vi "Filter OPC-UA-Items.vi"() -> ()   [LabVIEW 2016]
panel:
  out "Founf OPC Items":string[](array[string])
  out "found":i32
  in  "regular expression":string
  in  "sorted array":T1(array[cluster])
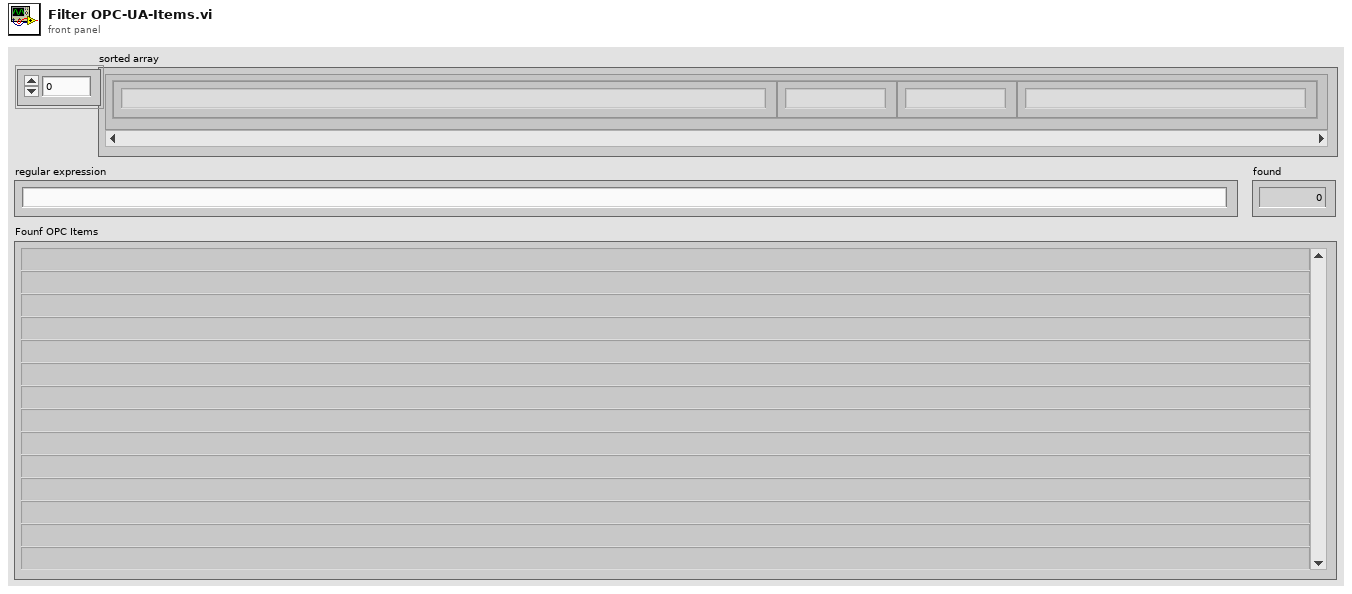
[diagram p1: front panel]
types:
  T1 = cluster{"node name":string, "String":string, "String":string, "node path":string}[]
  T2 = enum16{"open", "replace", "create", "open or create", "replace or create", "replace or create with confirmation"}
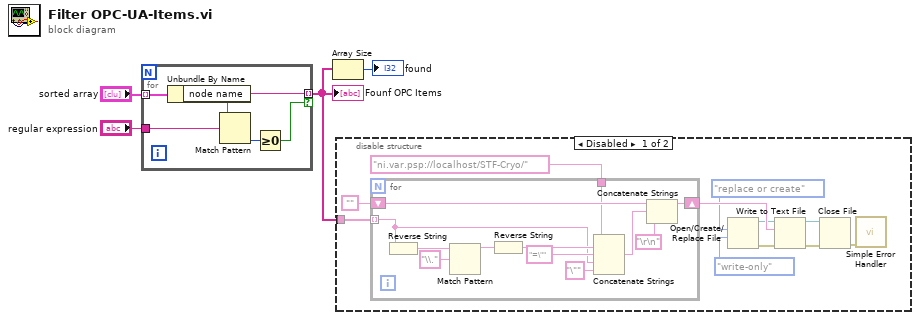
[diagram p0: block diagram]
diagram:
  n1 = for {
    tunnel: "sorted array" -> [w9] mode=indexing
    tunnel: "regular expression" -> [w8]
    tunnel: [w7] -> w1 mode=indexing if=w5
    n2 = Unbundle By Name(w9) -> ("node name"=w7:string)
    n3 = Match Pattern(string=w7, regular expression=w8) -> (offset past match=w6:i32)  [unwired: 1 in, 3 out]
    n4 = Greater Or Equal To 0?(x=w6) -> (x >= 0?=w5:bool)
  }
  "Founf OPC Items" <- w1
  n5 = Array Size(array=w1) -> (size(s)=→"found":i32)
  n6 = disable-structure shown="Disabled" {
    disable-tunnel: w1 -> [w19 _]
    frame Disabled {
      n7 = for {
        shift-right: [w31] -> w18
        shift-left: "" -> [w32]
        tunnel: w19 -> [w23] mode=indexing
        tunnel: "ni.var.psp://localhost/STF-Cryo/" -> [w26]
        n8 = Reverse String(1:w23) -> (0:w29:string)
        n9 = Match Pattern(string=w29, regular expression="\\.") -> (before substring=w28:string)  [unwired: 1 in, 3 out]
        n10 = Reverse String(1:w28) -> (0:w27:string)
        n11 = Concatenate Strings(w26, w27, "=\"" ("string"), w23, "\"" ("string")) -> (w25:string)
        n12 = Concatenate Strings(w32, w25, "\r\n") -> (w31:string)
      }
      n13 = Open/Create/Replace File(operation (0:open)=T2."replace or create", access (0:read/write)=enum16{"read/write", "read-only", "write-only"}."write-only") -> (refnum out=w14:refnum<file>, error out=w15:errorcluster)  [unwired: 4 in, 1 out]
      n14 = Write to Text File(file (use dialog)=w14, text=w18, error in=w15) -> (refnum out=w13:refnum<file>, error out=w12:errorcluster)  [unwired: 1 in, 1 out]
      n15 = Close File(refnum=w13, error in=w12) -> (error out=w11:errorcluster)  [unwired: 1 out]
      n16 = call <vilib>:"Simple Error Handler.vi"("error in (no error)"=w11) -> ()  [unwired: 4 in, 5 out]
    }
    frame Enabled {
    }
  }
